vi "Map.vi"(4 "Output High":dbl, 5 "Input High":dbl, 6 "Output Low":dbl, 7 "Input Low":dbl, 11 "Input":dbl) -> (3 "Output":dbl)   [LabVIEW 2015]
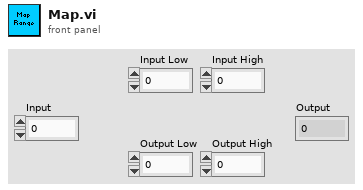
[diagram p1: front panel]
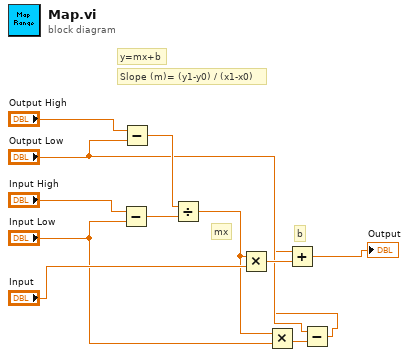
[diagram p0: block diagram]
diagram:
  # "b"
  # "mx"
  # "y=mx+b"
  # "Slope (m)= (y1-y0) / (x1-x0)"
  n1 = Subtract(x="Input High", y="Input Low") -> (x-y=w12:dbl)
  n2 = Subtract(x="Output High", y="Output Low") -> (x-y=w6:dbl)
  n3 = Divide(x=w6, y=w12) -> (x/y=w4:dbl)
  n4 = Multiply(x=w4, y="Input") -> (x*y=w11:dbl)
  n5 = Multiply(x=w4, y="Input Low") -> (x*y=w2:dbl)
  n6 = Subtract(x="Output Low", y=w2) -> (x-y=w1:dbl)
  n7 = Add(x=w1, y=w11) -> (x+y=→"Output":dbl)
